vi "GOMDBTS2048 substitution Get Date Time.vi"(8 "error in (no error)":errorcluster, 11 "handle":i32) -> (0 "error out":errorcluster, 1 "year":i32, 2 "month":i32, 3 "day":i32, 4 "mm":i32, 5 "hh":i32, 6 "function return":i32, 7 "ss":i32)   [LabVIEW 2015, in "GOMDBTS2048.lvlib"]
doc: "GOBTS2048DLL int __stdcall GOMDBTS2048_substitutionGetDateTime(int handle, int* day, int* month, int* year, int* hh, int* mm, int* ss);"
uses:
  GOMDBTS2048.lvlib
  runtime/GOMDBTS2048.dll
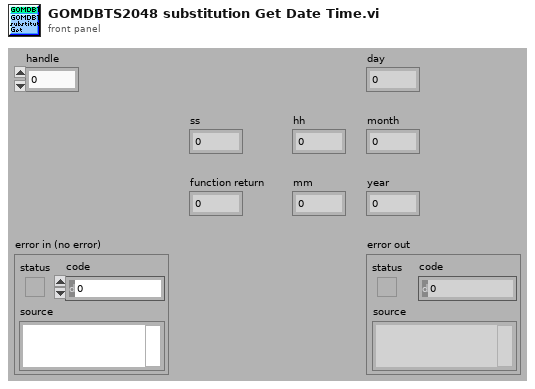
[diagram p1: front panel]
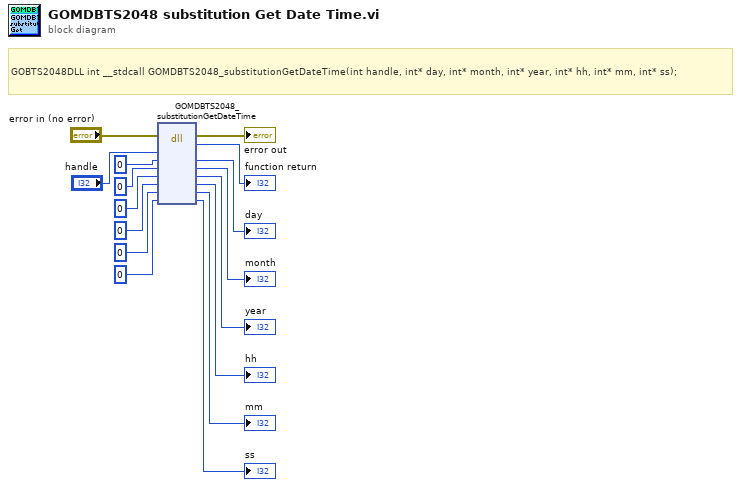
[diagram p0: block diagram]
diagram:
  # "GOBTS2048DLL int __stdcall GOMDBTS2048_substitutionGetDateTime(int handle, int* day, int* month, int* year, int* hh, int* mm, int* ss);"
  n1 = dll-call lib="C:/Users/rkoch/Documents/GO_Library/runtime/GOMDBTS2048.*" fn="GOMDBTS2048_substitutionGetDateTime"(error in="error in (no error)", "handle"="handle", "day"=0, "month"=0, "year"=0, "hh"=0, "mm"=0, "ss"=0) -> (error out=→"error out":errorcluster, →"function return":i32, "day"=→"day":i32, "month"=→"month":i32, "year"=→"year":i32, "hh"=→"hh":i32, "mm"=→"mm":i32, "ss"=→"ss":i32)  [unwired: 3 in, 1 out]
